vi "Trigger.vi"(0 "VISA IN":refnum<visa-resource-name>, 1 "Trigger Mode":string(combo)="HOLD", 5 "error in":errorcluster, 7 "Channel":i32) -> (14 "VISA Out":refnum<visa-resource-name>, 19 "error out":errorcluster)   [LabVIEW 2018, in "PNA-X.lvlib"]
doc: "SENSe<cnum>:SWEep:MODE <char> \n(Read-Write) Sets the number of trigger signals the specified channel will ACCEPT. \nSee Triggering the PNA Using SCPI. \nParameters \n<cnum> Any existing channel number. If unspecified, value is set to 1 \n<char> Trigger mode. Choose from: \nHOLD - channel will not trigger \nCONTinuous - channel triggers indefinitely \nGROups - channel accepts the number of triggers specified with the last \nSENS:SWE:GRO:COUN <num>. This is one of the PNA overlapped commands. Learn \nmore. \nHow to specify Single Trigger - Internal or External: \n1. Send SENS:SWE:GRO:COUN 1 \n2. Send SENS:SWE:MODE GROups. When received, the specified PNA channel \nIMMEDIATELY accepts one trigger signal, if available, then goes into hold. To accept \nanother trigger signal, resend SENS:SWE:MODE GROups. \n1817\n\nExamples SENS:SWE:MODE CONT \nsense2:sweep:mode hold \nQuery Syntax SENSe<cnum>:SWEep:MODE? \nReturn Type Character \nDefault CONTinuous"
uses:
  PNA-X.lvlib
panel:
  in  "Groups Count":i32
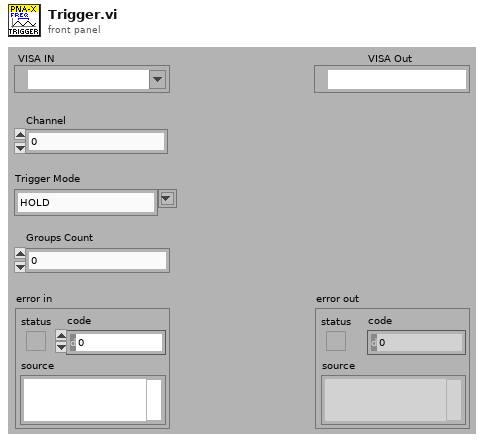
[diagram p1: front panel]
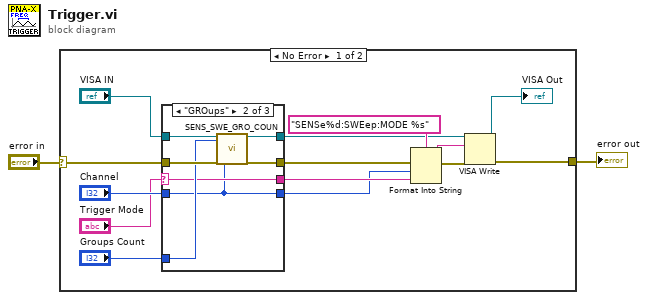
[diagram p0: block diagram]
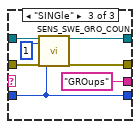
[diagram p3: hidden frame]
diagram:
  n1 = case shown="No Error" "error in" {
    selector: "error in" -> [w8 w35]
    tunnel: [w16 w35] -> w1
    frame No Error {
      n2 = case shown="\"GROups\"" "Trigger Mode" {
        selector: "Trigger Mode" -> [w18 w22 _]
        tunnel: [w20 w24 w33] -> w11
        tunnel: "VISA IN" -> [w20 w25 w32]
        tunnel: "Channel" -> [w17 w21 w28]
        tunnel: w8 -> [w19 w27 w31]
        tunnel: [w19 w26 w30] -> w7
        tunnel: [w18 w22 "GROups"] -> w5
        tunnel: "Groups Count" -> [_ w23 _]
        tunnel: [w17 w21 w28] -> w3
        frame Default {
        }
        frame "GROups" {
          n3 = call "SENS_SWE_GRO_COUN.vi"("VISA IN"=w25, "Count"=w23, "error in"=w27, "Channel"=w21) -> ("VISA Out"=w24:refnum<visa-resource-name>, "error out"=w26:errorcluster)  [unwired: 14 in]
        }
        frame "SINGle" {
          n4 = call "SENS_SWE_GRO_COUN.vi"("VISA IN"=w32, "Count"=1, "error in"=w31, "Channel"=w28) -> ("VISA Out"=w33:refnum<visa-resource-name>, "error out"=w30:errorcluster)  [unwired: 14 in]
        }
      }
      n5 = Format Into String(format string="SENSe%d:SWEep:MODE %s" ("Cmdline"), error in=w7, w3, w5) -> (resulting string=w13:string, error out=w14:errorcluster)  [unwired: 1 in]
      n6 = VISA Write(VISA resource name=w11, write buffer=w13, error in (no error)=w14) -> (VISA resource name out=→"VISA Out":refnum<visa-resource-name>, error out=w16:errorcluster)  [unwired: 1 out]
    }
    frame Error {
    }
  }
  "error out" <- w1
